vi "Read Data.vi"(8 "error in":errorcluster, 11 "PAS in":refnum<class "PAS.lvclass">) -> (0 "error out":errorcluster, 2 "PAS Data.lvclass":refnum<class "PAS Data.lvclass">, 3 "PAS out":refnum<class "PAS.lvclass">)   [LabVIEW 2015, in "PAS.lvclass"]
uses:
  PAS.lvclass
  Data/Main/PAS Data.lvclass
  PAS.lvclass/PAS.ctl
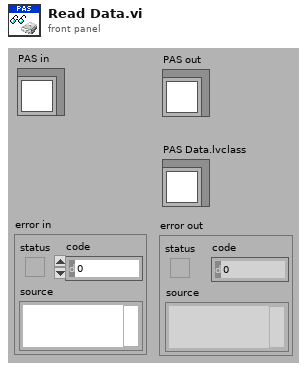
[diagram p1: front panel]
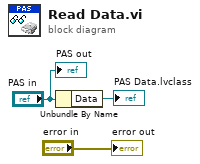
[diagram p0: block diagram]
diagram:
  n1 = Unbundle By Name("PAS in") -> ("Data"=→"PAS Data.lvclass":refnum<class "PAS Data.lvclass">)
  "error out" <- "error in"
  "PAS out" <- "PAS in"
